vi "Caption - Get.vi"() -> ()   [LabVIEW 2013]
panel:
  out "Label.Text":string[](array[string])
  out "Ref":refnum<vi>[](array[refnum])
  out "Caption":T1(array[cluster])
  in  "Get/Set":bool
  in  "vi path":path
  # "lšeg‰šN"
  # "°e RaW"
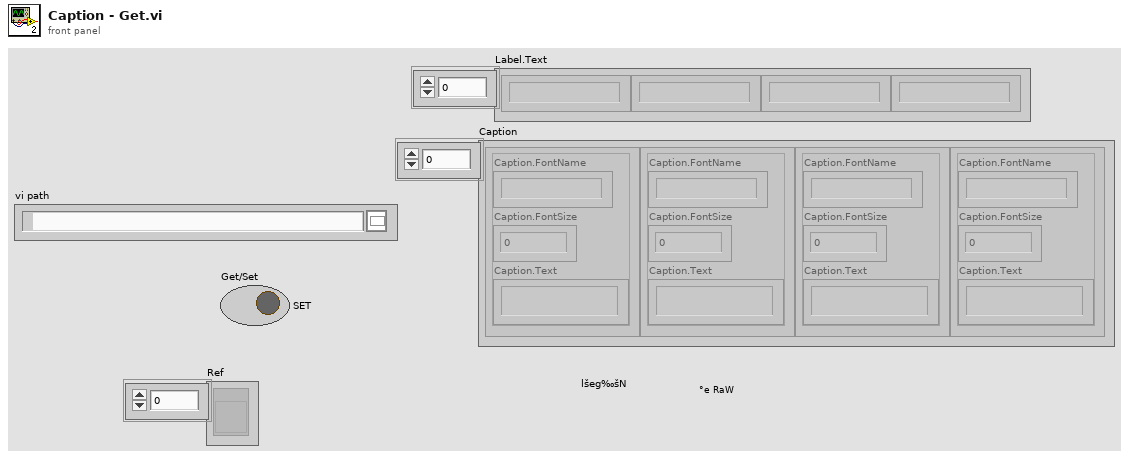
[diagram p1: front panel]
types:
  T1 = cluster{"Caption.FontName":string, "Caption.FontSize":u32, "Caption.Text":string}[]
  T2 = cluster{"Caption.FontName":string, "Caption.FontSize":u32, "Caption.Text":string}
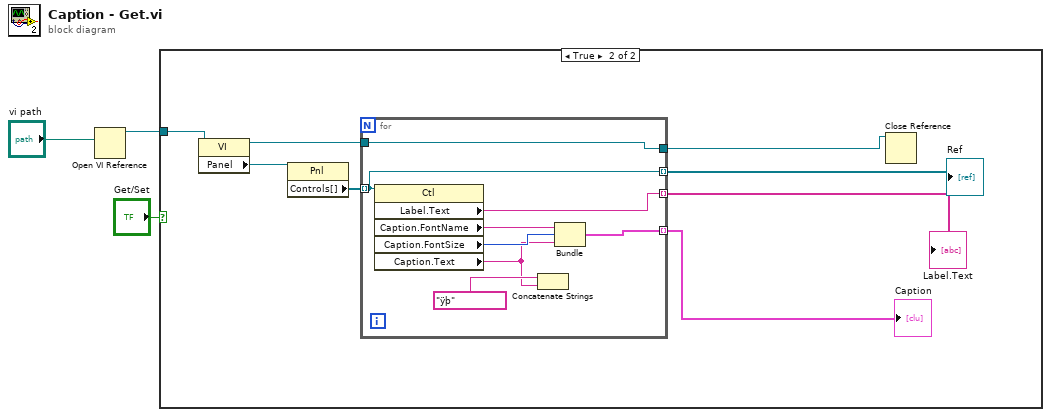
[diagram p0: block diagram]
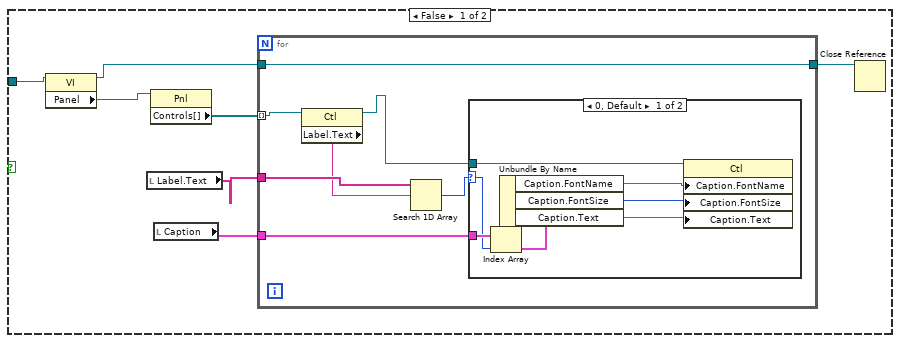
[diagram p2: hidden frame]
diagram:
  n1 = Open VI Reference(vi path="vi path") -> (vi reference=w3:refnum<vi>)  [unwired: 5 in, 1 out]
  n2 = case shown="True" "Get/Set" {
    tunnel: w3 -> [w10 w32]
    frame False {
      n3 = property class="VI"(reference=w10) -> (reference out=w5:refnum<vi>, "Panel"=w9:refnum<vi>)  [unwired: 1 in, 1 out]
      n4 = local read "Label.Text"() -> (w7:string[])
      n5 = property class="Pnl"(reference=w9) -> ("Controls[]"=w8:refnum<vi>[])  [unwired: 1 in, 2 out]
      n6 = local read "Caption"() -> (w6:T1)
      n7 = for {
        tunnel: w8 -> [w17] mode=indexing
        tunnel: w7 -> [w16]
        tunnel: w6 -> [w13]
        tunnel: w5 -> [w11]
        tunnel: [w11] -> w4
        n8 = property class="Ctl"(reference=w17) -> (reference out=w12:refnum<vi>, "Label.Text"=w15:string)  [unwired: 1 in, 1 out]
        n9 = Search 1D Array(1D array=w16, element=w15) -> (index of element=w14:i32)  [unwired: 1 in]
        n10 = case shown="0, Default" w14 {
          selector: w14 -> [w23 _]
          tunnel: w13 -> [w24 _]
          tunnel: w12 -> [w18 _]
          frame 0, Default {
            n11 = Index Array(array=w24, index=w23) -> (element=w22:T2)
            n12 = Unbundle By Name(w22) -> ("Caption.FontName"=w21:string, "Caption.FontSize"=w20:u32, "Caption.Text"=w19:string)
            n13 = property class="Ctl"(reference=w18, "Caption.FontName"=w21, "Caption.FontSize"=w20, "Caption.Text"=w19) -> ()  [unwired: 1 in, 2 out]
          }
          frame -1 {
          }
        }
      }
      n14 = Close Reference(reference=w4) -> ()  [unwired: 1 in, 1 out]
    }
    frame True {
      n15 = property class="VI"(reference=w32) -> (reference out=w28:refnum<vi>, "Panel"=w31:refnum<vi>)  [unwired: 1 in, 1 out]
      n16 = property class="Pnl"(reference=w31) -> ("Controls[]"=w30:refnum<vi>[])  [unwired: 1 in, 2 out]
      n17 = for {
        tunnel: w30 -> [w35] mode=indexing
        tunnel: [w38] -> w27 mode=indexing
        tunnel: [w37] -> w29
        tunnel: w28 -> [w37]
        tunnel: [w36] -> w25 mode=indexing
        tunnel: [w35] -> w26 mode=indexing
        n18 = property class="Ctl"(reference=w35) -> ("Label.Text"=w36:string, "Caption.FontName"=w40:string, "Caption.FontSize"=w39:u32, "Caption.Text"=w33:string)  [unwired: 1 in, 2 out]
        n19 = Concatenate Strings("ÿþ", w33) -> ()  [unwired: 1 out]
        n20 = Bundle("Caption.FontName"=w40, "Caption.FontSize"=w39, "Caption.Text"=w33) -> (w38:T2)  [unwired: 1 in]
      }
      "Caption" <- w27
      "Ref" <- w26
      "Label.Text" <- w25
      n21 = Close Reference(reference=w29) -> ()  [unwired: 1 in, 1 out]
    }
  }
